vi "AuxNetwork.vi"   [LabVIEW 2020]
uses:
  AuxGlobals.vi
  <vilib>/Rock Robotics/Network Tables/NT Write Number.vi
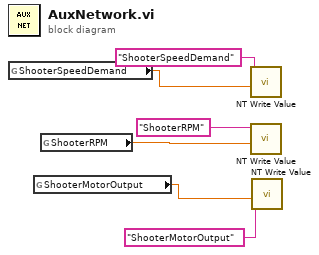
[diagram p0: block diagram]
diagram:
  n1 = global read "AuxGlobals.vi" "ShooterSpeedDemand"() -> (w1:dbl)
  n2 = global read "AuxGlobals.vi" "ShooterMotorOutput"() -> (w3:dbl)
  n3 = global read "AuxGlobals.vi" "ShooterRPM"() -> (w2:dbl)
  n4 = call-poly <vilib>:"NT Write Value.vi"("Numeric"=w1, "Name"="ShooterSpeedDemand") -> ()  [unwired: 9 in, 1 out]
  n5 = call-poly <vilib>:"NT Write Value.vi"("Numeric"=w2, "Name"="ShooterRPM") -> ()  [unwired: 9 in, 1 out]
  n6 = call-poly <vilib>:"NT Write Value.vi"("Numeric"=w3, "Name"="ShooterMotorOutput") -> ()  [unwired: 9 in, 1 out]
